vi "List State.vi"(8 "error in (no error)":errorcluster, 9 "Enable List Trigger (F)":bool, 10 "Enable List State (F)":bool, 11 "VISA resource name":refnum<visa-resource-name>) -> (0 "error out":errorcluster, 3 "VISA resource name out":refnum<visa-resource-name>)   [LabVIEW 2017, in "HH PLI Series.lvlib"]
doc: "Initiates a programmed list.\n\n<b>Note</b>\nUse VI \"Configure List\" to define a couple of list points.\nUse VI \"Configure Input\" to enable or disable instrument input."
uses:
  HH PLI Series.lvlib
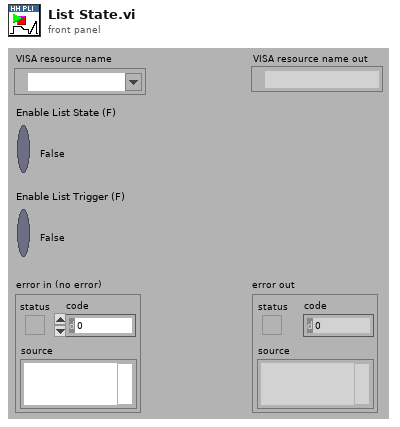
[diagram p1: front panel]
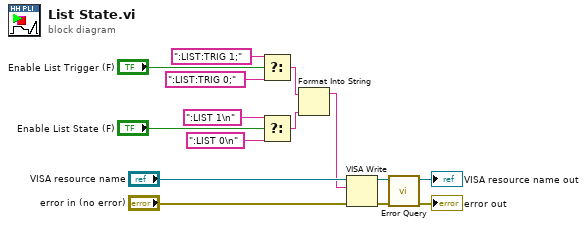
[diagram p0: block diagram]
diagram:
  n1 = Select(t=":LIST:TRIG 1;", s="Enable List Trigger (F)", f=":LIST:TRIG 0;") -> (s? t:f=w1:string)
  n2 = Select(t=":LIST 1\n", s="Enable List State (F)", f=":LIST 0\n") -> (s? t:f=w2:string)
  n3 = Format Into String(initial string=w1, w2) -> (resulting string=w3:string)  [unwired: 2 in, 1 out]
  n4 = VISA Write(VISA resource name="VISA resource name", write buffer=w3, error in (no error)="error in (no error)") -> (VISA resource name out=w12:refnum<visa-resource-name>, error out=w13:errorcluster)  [unwired: 1 out]
  n5 = call "Error Query.vi"("error in (no error)"=w13, "VISA resource name"=w12) -> ("error out"=→"error out":errorcluster, "VISA resource name out"=→"VISA resource name out":refnum<visa-resource-name>)  [unwired: 6 in, 2 out]
